vi "save.vi"(6 "Save data":bool, 9 "String":string, 10 "Array":dbl[][](array[numeric]), 11 "File_name":path) -> ()   [LabVIEW 2020]
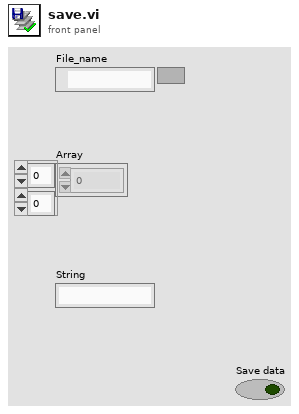
[diagram p1: front panel]
types:
  T1 = enum16{"open", "replace", "create", "open or create", "replace or create", "replace or create with confirmation"}
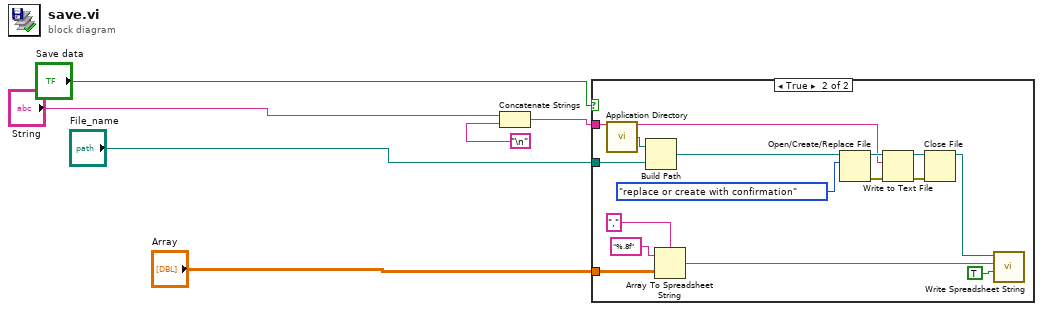
[diagram p0: block diagram]
diagram:
  n1 = Concatenate Strings("String", "\n") -> (w2:string)
  n2 = case shown="True" "Save data" {
    tunnel: w2 -> [_ w10]
    tunnel: "File_name" -> [_ w9]
    tunnel: "Array" -> [_ w8]
    frame False {
    }
    frame True {
      n3 = call <vilib>:"Application Directory.vi"() -> ("Application Directory"=w19:path)
      n4 = Build Path(base path=w19, name or relative path=w9) -> (appended path=w18:path)
      n5 = Array To Spreadsheet String(delimiter (Tab)=",", array=w8, 3:"%.8f" ("format string")) -> (spreadsheet string=w7:string)
      n6 = Open/Create/Replace File(file path (use dialog)=w18, operation (0:open)=T1."replace or create with confirmation") -> (refnum out=w14:refnum<file>, error out=w13:errorcluster)  [unwired: 4 in, 1 out]
      n7 = Write to Text File(file (use dialog)=w14, text=w10, error in=w13) -> (refnum out=w12:refnum<file>, error out=w11:errorcluster)  [unwired: 1 in, 1 out]
      n8 = Close File(refnum=w12, error in=w11) -> (path=w17:path)  [unwired: 1 out]
      n9 = call <vilib>:"Write Spreadsheet String.vi"("append to file? (new file:F)"=TRUE, "spreadsheet string"=w7, "file path (dialog if empty)"=w17) -> ()  [unwired: 7 in, 2 out]
    }
  }
